vi "Trafik lambası simülatörü.vi"() -> ()   [LabVIEW 2014]
panel:
  in  "stop":bool
  in  "Yeşilin Süresi":dbl
  in  "Sarının Süresi":dbl
  in  "Kırmızı Süresi":dbl
  out "Yeşil":bool
  out "Sarı":bool
  out "Kırmızı":bool
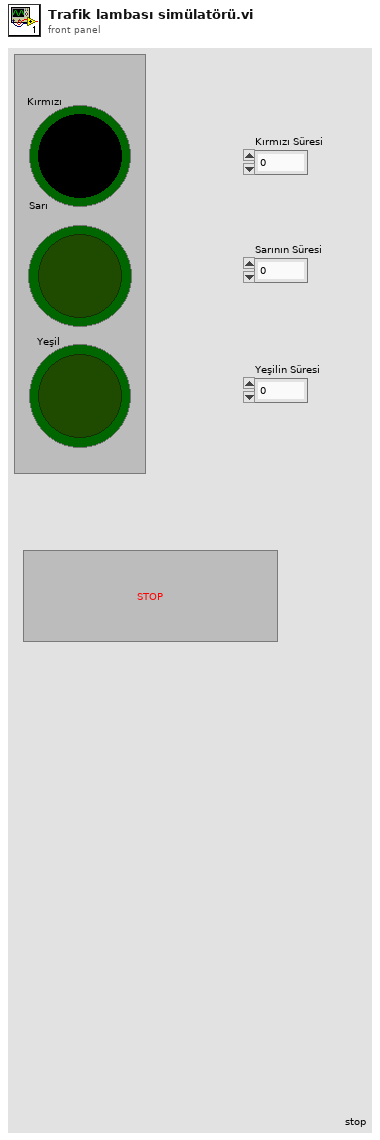
[diagram p1: front panel]
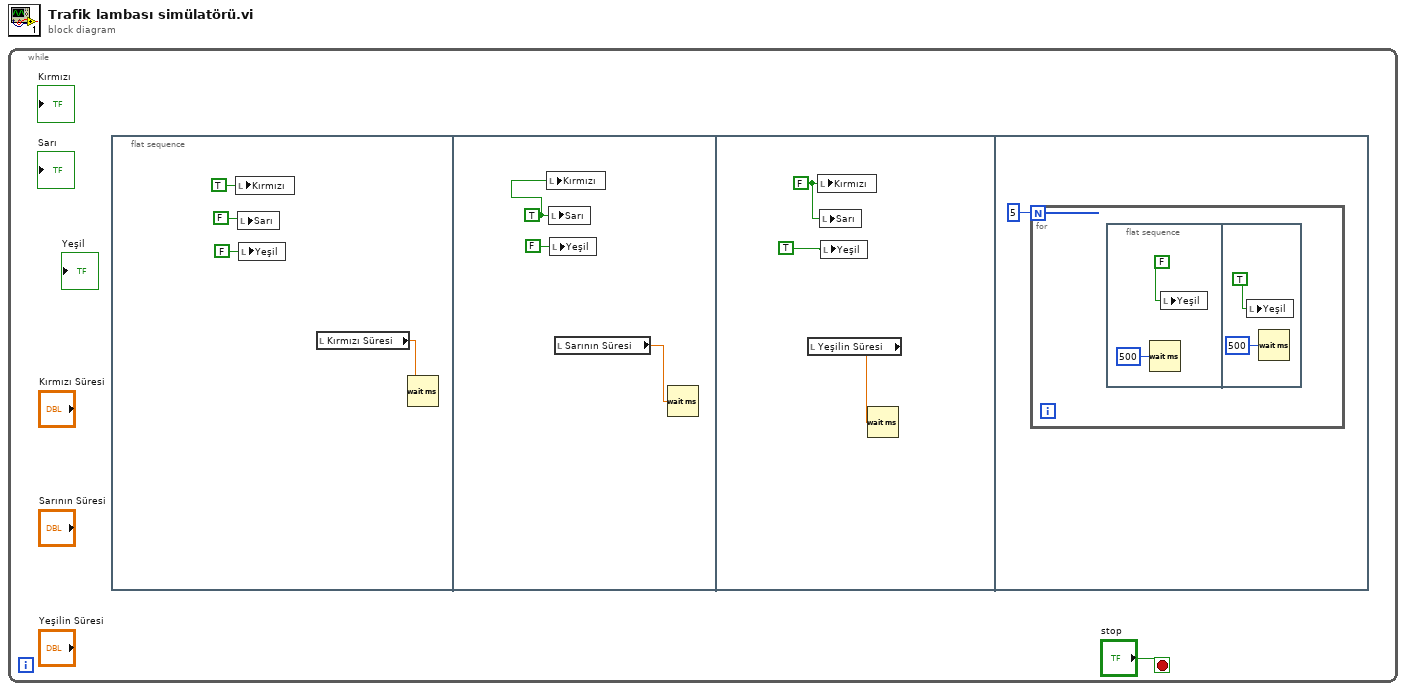
[diagram p0: block diagram]
diagram:
  n1 = while {
    stop <- "stop" stop-if-true
    n2 = flat-sequence {
      frame #0 {
        n3 = local write "Kırmızı"(TRUE ("Kırmızı")) -> ()
        n4 = local write "Sarı"(FALSE ("Sarı")) -> ()
        n5 = local write "Yeşil"(FALSE ("Yeşil")) -> ()
        n6 = local read "Kırmızı Süresi"() -> (w2:dbl)
        n7 = Wait (ms)(milliseconds to wait=w2) -> ()  [unwired: 1 out]
      }
      frame #1 {
        w7 = TRUE ("Sarı")
        n8 = local write "Kırmızı"(w7) -> ()
        n9 = local write "Sarı"(w7) -> ()
        n10 = local write "Yeşil"(FALSE ("Yeşil")) -> ()
        n11 = local read "Sarının Süresi"() -> (w6:dbl)
        n12 = Wait (ms)(milliseconds to wait=w6) -> ()  [unwired: 1 out]
      }
      frame #2 {
        w9 = FALSE ("Kırmızı")
        n13 = local read "Yeşilin Süresi"() -> (w11:dbl)
        n14 = local write "Kırmızı"(w9) -> ()
        n15 = local write "Sarı"(w9) -> ()
        n16 = local write "Yeşil"(TRUE) -> ()
        n17 = Wait (ms)(milliseconds to wait=w11) -> ()  [unwired: 1 out]
      }
      frame #3 {
        n18 = for {
          N: 5 -> [_]
          n19 = flat-sequence {
            frame #0 {
              n20 = Wait (ms)(milliseconds to wait=u32 500) -> ()  [unwired: 1 out]
              n21 = local write "Yeşil"(FALSE) -> ()
            }
            frame #1 {
              n22 = local write "Yeşil"(TRUE) -> ()
              n23 = Wait (ms)(milliseconds to wait=u32 500) -> ()  [unwired: 1 out]
            }
          }
        }
      }
    }
  }
